vi "Teleop.vi"(10 "Match Info":T1={"Autonomous Elapsed Seconds"=0.0, "TeleOp Elapsed Seconds"=0.0, "Disabled Elapsed Seconds"=0.0, "Visited Autonomous"=FALSE, "Visited TeleOp"=FALSE, "Visited Disabled"=FALSE, "Autonomous Settings"={"Autonomous Style"=enum."Independent", "VI Refnum"=refnum}}, 11 "Call Context":T2) -> ()   [LabVIEW 2015]
doc: "This VI is called for each TeleOp packet received from the DS where the robot is not disabled. It is often used to read from the joysticks and update I/O or to update setpoints for timed control loops. It should complete and return within 20 milliseconds or it may miss DS packets."
uses:
  <vilib>/Rock Robotics/WPI/DriverStation/WPI_DriverStationDerivedRobotMode.ctl
  <vilib>/Rock Robotics/WPI/DriverStation/WPI_DriverStationMatch Info.ctl
  <vilib>/Rock Robotics/WPI/Utilities/WPI_GetSetVariantRefNum.vi
  <vilib>/Rock Robotics/Network Tables/NT Write Boolean Array.vi
  <vilib>/Rock Robotics/Network Tables/NT Write Numeric Array.vi
  <vilib>/Rock Robotics/Network Tables/NT Read Boolean.vi
  <vilib>/Rock Robotics/Network Tables/NT Read Number.vi
  <vilib>/Rock Robotics/Network Tables/NT Write Boolean.vi
  <vilib>/Rock Robotics/Network Tables/NT Write Number.vi
panel:
  out "Low Switch":bool
  out "High Switch":bool
  out "POT Sensor Meter":dbl(knob) scale=78.0..98.0
  out "POT Sensor Value":dbl
  out "Sample Slider 0":dbl(slide) scale=0.0..5.0
  out "Sample Boolean 1":bool
  out "Sample Boolean 0":bool
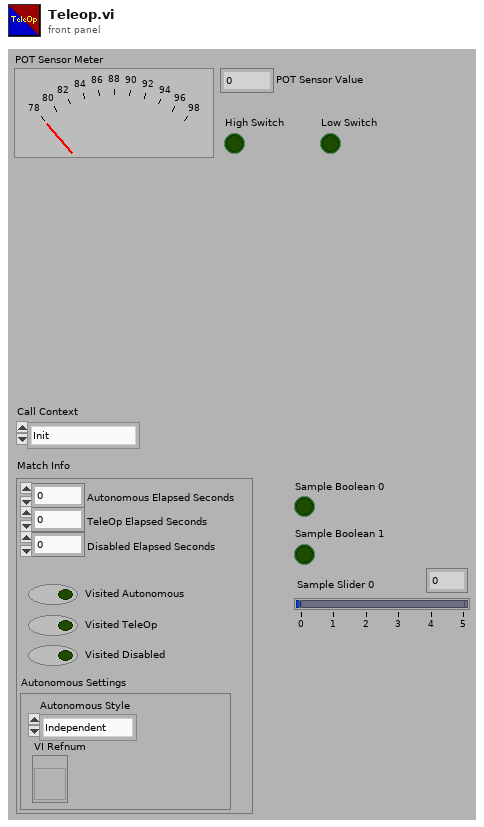
[diagram p1: front panel]
types:
  T1 = typedef "WPI_DriverStationMatch Info.ctl" = cluster{"Autonomous Elapsed Seconds":dbl, "TeleOp Elapsed Seconds":dbl, "Disabled Elapsed Seconds":dbl, "Visited Autonomous":bool, "Visited TeleOp":bool, "Visited Disabled":bool, "Autonomous Settings":cluster{"Autonomous Style":enum16{"Iterative", "Independent"}, "VI Refnum":refnum<vi>}}
  T2 = typedef "WPI_DriverStationDerivedRobotMode.ctl" = enum16{"Init", "Execute", "Stop"}
  T3 = typedef "WPI_JoystickDevRef.ctl" = cluster{"Device":T4}
  T4 = typedef "WPI_JoystickDeviceEnum.ctl" = enum16{"USB 0", "USB 1", "USB 2", "USB 3", "USB 4", "USB 5"}
  T5 = typedef "WPI_SwitchDevRef.ctl" = cluster{"DevStatus":errorcluster, "DIO Channel":T6, "CntIndex":T7, "Normally Closed":bool}
  T6 = typedef "FPGA_DIOChannel.ctl" = enum8{"DIO 0", "DIO 1", "DIO 2", "DIO 3", "DIO 4", "DIO 5", "DIO 6", "DIO 7", "DIO 8", "DIO 9", "DIO MXP 0", "DIO MXP 1", "DIO MXP 2", "DIO MXP 3", "DIO MXP 4", "DIO MXP 5", "DIO MXP 6", "DIO MXP 7", "DIO MXP 8", "DIO MXP 9", "DIO MXP 10", "DIO MXP 11", "DIO MXP 12", "DIO MXP 13", "DIO MXP 14", "DIO MXP 15", "Invalid"}
  T7 = typedef "FPGA_CounterCtrSystemIndex.ctl" = enum8{"Ctr 0", "Ctr 1", "Ctr 2", "Ctr 3", "Ctr 4", "Ctr 5", "Ctr 6", "Ctr 7", "Invalid"}
  T8 = cluster{"Axes[0]":dbl, "Axes[1]":dbl, "Axes[2]":dbl, "Axes[3]":dbl, "Axes[4]":dbl, "Axes[5]":dbl, "Axes[6]":dbl, "Axes[7]":dbl, "Axes[8]":dbl}
  T9 = typedef "WPI_RobotDriveDevRef.ctl" = cluster{"DevStatus":errorcluster, "Motors[]":T10[], "Square Inputs":bool, "Max Output":dbl}
  T10 = typedef "WPI_MotorControlDeviceRef.ctl" = cluster{"DeviceStatus":errorcluster, "Type":T11, "PWM":cluster{"PWM Channel":T12, "DeadBand":T13}, "CAN":cluster{"Device Number":u8, "Control Mode":T14, "Semaphore":T15, "Max Vout":dbl, "TalonSRX Control Mode":T16}, "Invert":bool}
  T11 = typedef "WPI_MotorControlType.ctl" = enum16{"PWM", "CAN", "CANTalonSRX"}
  T12 = typedef "FPGA_DIOPWMChannel.ctl" = enum8{"PWM 0", "PWM 1", "PWM 2", "PWM 3", "PWM 4", "PWM 5", "PWM 6", "PWM 7", "PWM 8", "PWM 9", "PWM MXP 0", "PWM MXP 1", "PWM MXP 2", "PWM MXP 3", "PWM MXP 4", "PWM MXP 5", "PWM MXP 6", "PWM MXP 7", "PWM MXP 8", "PWM MXP 9", "Invalid"}
  T13 = typedef "WPI_PWMDeadband.ctl" = cluster{"Name":string, "maxPositivePwm":i32, "minPositivePwm":i32, "centerPwm":i32, "maxNegativePwm":i32, "minNegativePwm":i32, "angularRange":u16}
  T14 = typedef "WPI_CANJaguar_ControlMode.ctl" = enum8{"Percent VBus", "Current", "Speed", "Position", "Voltage"}
  T15 = typedef "Semaphore RefNum" = refnum<k1>
  T16 = typedef "WPI_CANTalonSRX_APIControlMode.ctl" = enum8{"Percent VBus", "Speed", "Position", "Slave", "Unchanged / Invalid", "Voltage Compensation", "Current", "Motion Profile"}
  T17 = cluster{"Buttons[0]":bool, "Buttons[1]":bool, "Buttons[2]":bool, "Buttons[3]":bool, "Buttons[4]":bool, "Buttons[5]":bool, "Buttons[6]":bool, "Buttons[7]":bool, "Buttons[8]":bool}
  T18 = typedef "WPI_PotentiometerDevRef.ctl" = cluster{"DevStatus":errorcluster, "Analog Channel":T19, "Invert Output":bool}
  T19 = typedef "FPGA_AIChannel.ctl" = enum8{"AI 0", "AI 1", "AI 2", "AI 3", "AI MXP 0", "AI MXP 1", "AI MXP 2", "AI MXP 3", "Invalid"}
  T20 = typedef "WPI_ServoDeviceRef.ctl" = cluster{"DeviceStatus":errorcluster, "PWM Channel":T12, "DeadBand":T13}
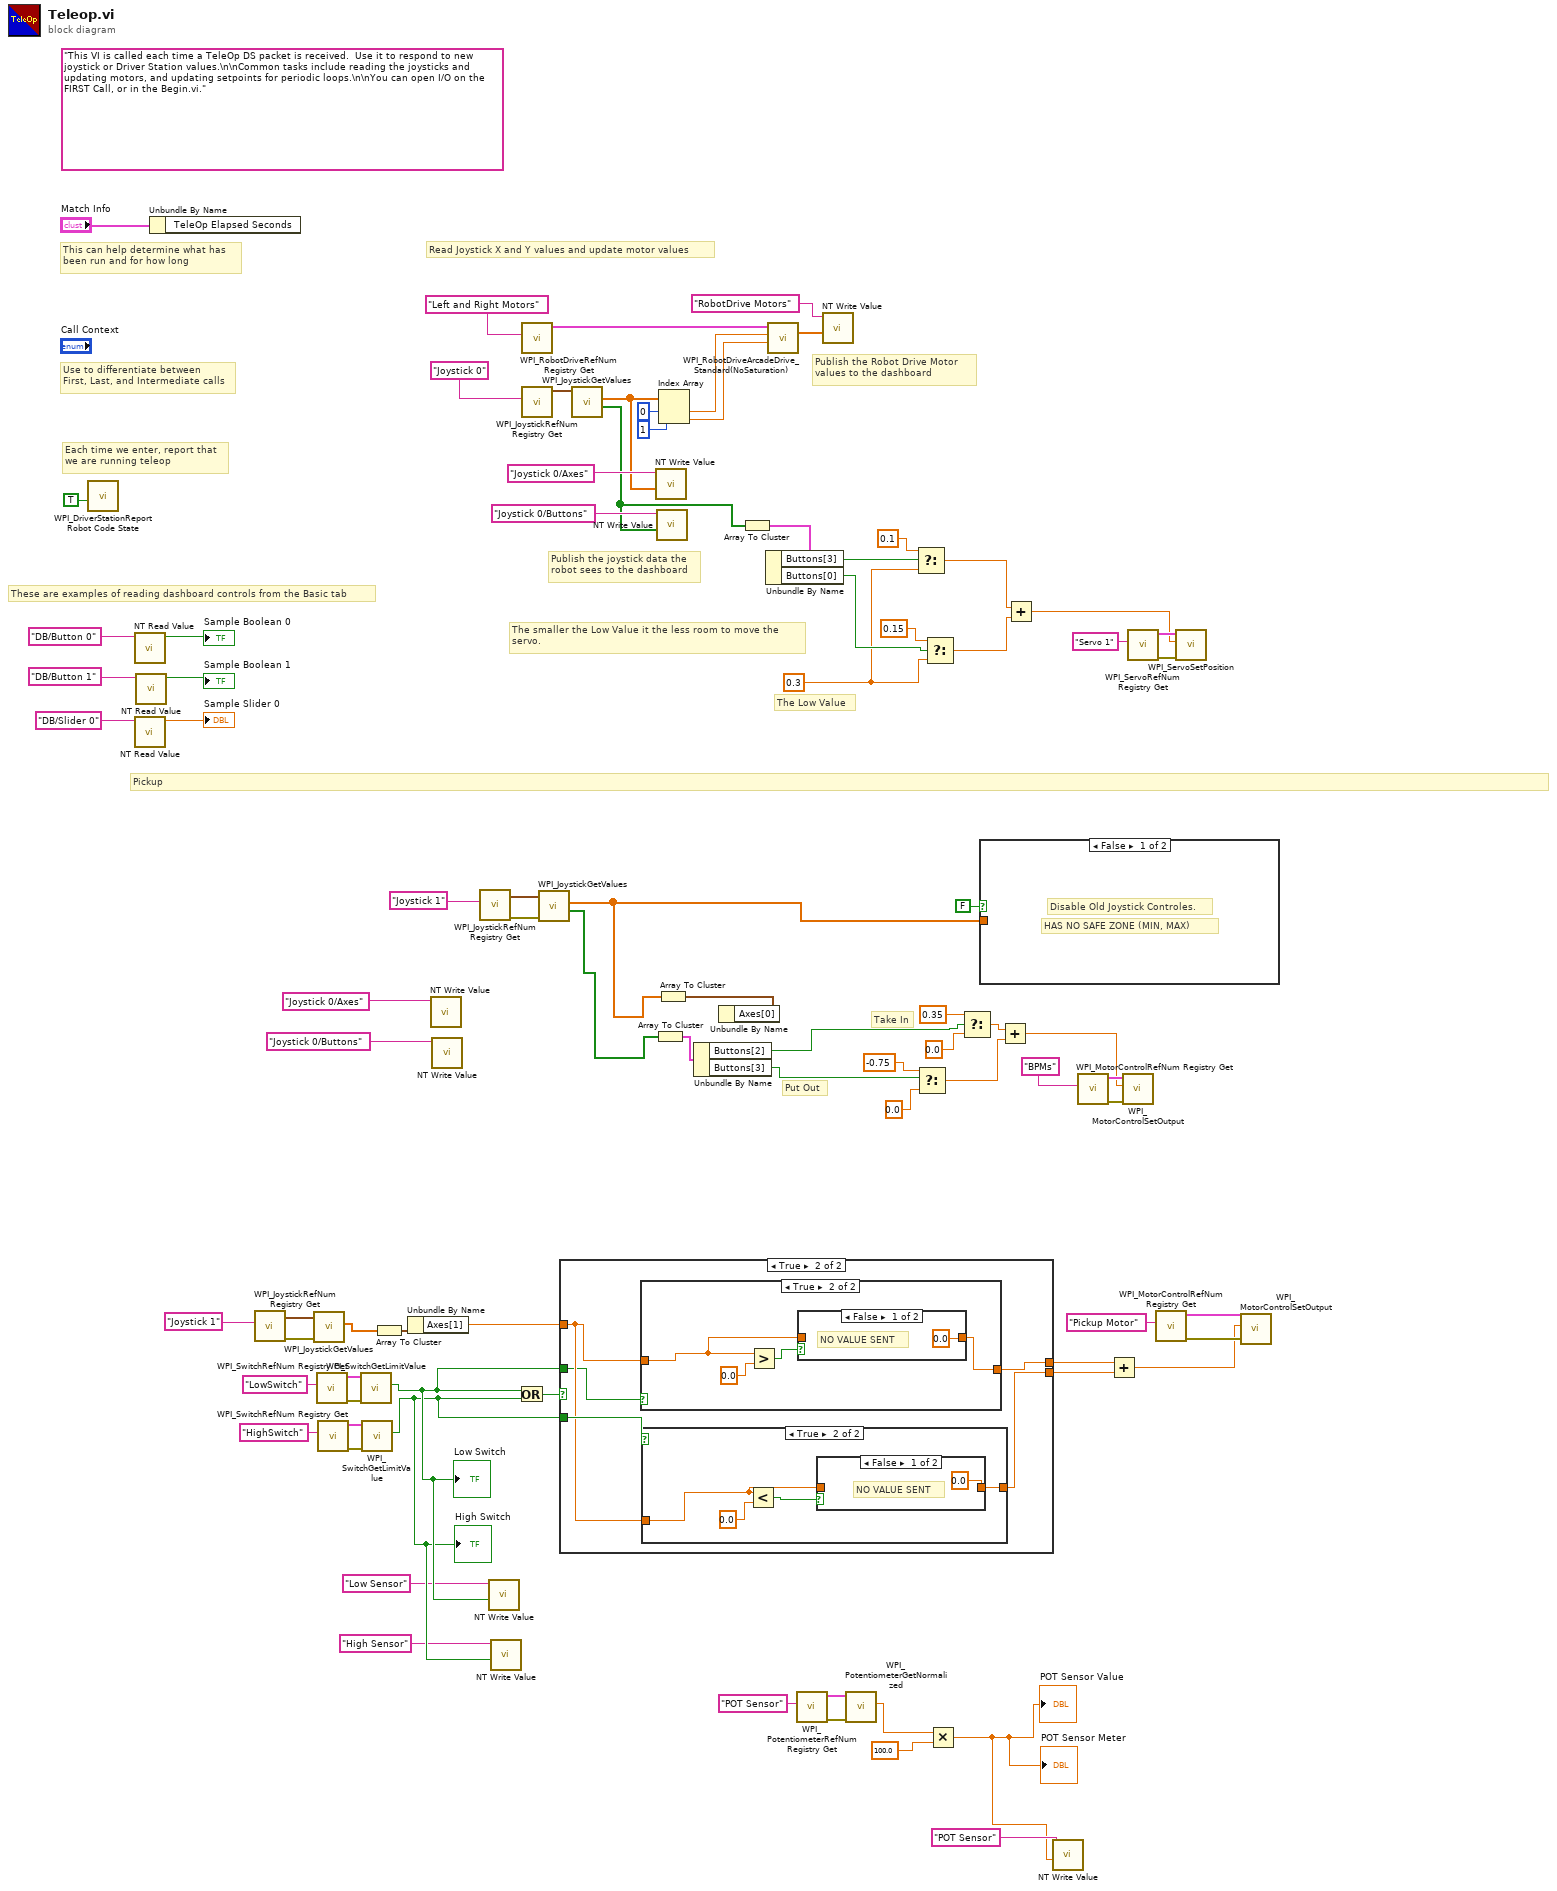
[diagram p0: block diagram]
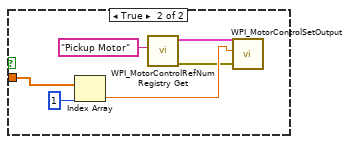
[diagram p2: hidden frame]
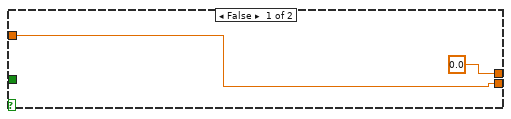
[diagram p3: hidden frame]
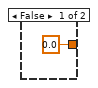
[diagram p4: hidden frame]
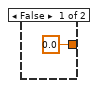
[diagram p6: hidden frame]
diagram:
  w1 = 0.3 ("f")
  (unwired) "This VI is called each time a TeleOp DS packet is received.  Use it to respond to new joystick or Driver Station values.\n\nCommon tasks include reading the joysticks and updating motors, and updating setpoints for periodic loops.\n\nYou can open I/O on the FIRST Call, or in the Begin.vi."
  # "The smaller the Low Value it the less room to move the \nservo."
  # "Put Out"
  # "Take In"
  # "The Low Value"
  # "Pickup"
  # "These are examples of reading dashboard controls from the Basic tab"
  # "Publish the Robot Drive Motor\nvalues to the dashboard"
  # "Publish the joystick data the\nrobot sees to the dashboard"
  # "Each time we enter, report that\nwe are running teleop"
  # "Use to differentiate between\nFirst, Last, and Intermediate calls"
  # "This can help determine what has\nbeen run and for how long"
  # "Read Joystick X and Y values and update motor values"
  n1 = call <vilib>:"WPI_DriverStationReport Robot Code State.vi"("TeleOp"=TRUE ("Autonomous")) -> ()  [unwired: 10 in, 1 out]
  n2 = call-poly <vilib>:"NT Read Value.vi"("Name"="DB/Button 0" ("refnum name")) -> ("Boolean"=→"Sample Boolean 0":bool)  [unwired: 9 in, 1 out]
  n3 = call-poly <vilib>:"NT Read Value.vi"("Name"="DB/Slider 0" ("refnum name")) -> ("Numeric"=→"Sample Slider 0":dbl)  [unwired: 9 in, 1 out]
  n4 = call-poly <vilib>:"NT Read Value.vi"("Name"="DB/Button 1" ("refnum name")) -> ("Boolean"=→"Sample Boolean 1":bool)  [unwired: 9 in, 1 out]
  n5 = Unbundle By Name("Match Info") -> ()  [unwired: 1 out]
  n6 = call <vilib>:"WPI_JoystickRefNum Registry Get.vi"("refnum name"="Joystick 1") -> ("error out"=w27:errorcluster, "JoystickDevRef"=w28:T3)  [unwired: 9 in]
  n7 = call <vilib>:"WPI_JoystickGetValues.vi"("error in (no error)"=w27, "JoystickDevRef"=w28) -> ("Axes"=w26:dbl[])  [unwired: 5 in, 4 out]
  n8 = call <vilib>:"WPI_SwitchRefNum Registry Get.vi"("refnum name"="LowSwitch") -> ("error out"=w34:errorcluster, "SwitchDevRef"=w35:T5)  [unwired: 9 in]
  n9 = call <vilib>:"WPI_SwitchRefNum Registry Get.vi"("refnum name"="HighSwitch") -> ("error out"=w31:errorcluster, "SwitchDevRef"=w32:T5)  [unwired: 9 in]
  n10 = call <vilib>:"WPI_SwitchGetLimitValue.vi"("error in (no error)"=w34, "SwitchDevRef"=w35) -> ("Switch Pressed"=w11:bool)  [unwired: 7 in, 2 out]
  "Low Switch" <- w11
  n11 = call <vilib>:"WPI_SwitchGetLimitValue.vi"("error in (no error)"=w31, "SwitchDevRef"=w32) -> ("Switch Pressed"=w10:bool)  [unwired: 7 in, 2 out]
  "High Switch" <- w10
  n12 = Array To Cluster(array=w26) -> (cluster=w25:T8)
  n13 = Unbundle By Name(w25) -> ("Axes[1]"=w24:dbl)
  n14 = call-poly <vilib>:"NT Write Value.vi"("Name"="Joystick 0/Axes") -> ()  [unwired: 10 in, 1 out]
  n15 = call-poly <vilib>:"NT Write Value.vi"("Name"="Joystick 0/Buttons") -> ()  [unwired: 10 in, 1 out]
  n16 = call <vilib>:"WPI_JoystickRefNum Registry Get.vi"("refnum name"="Joystick 1") -> ("error out"=w63:errorcluster, "JoystickDevRef"=w64:T3)  [unwired: 9 in]
  n17 = call-poly <vilib>:"NT Write Value.vi"("Boolean"=w11, "Name"="Low Sensor") -> ()  [unwired: 9 in, 1 out]
  n18 = call-poly <vilib>:"NT Write Value.vi"("Boolean"=w10, "Name"="High Sensor") -> ()  [unwired: 9 in, 1 out]
  n19 = Or(x=w11, y=w10) -> (x .or. y?=w36:bool)
  n20 = call <vilib>:"WPI_RobotDriveRefNum Registry Get.vi"("refnum name"="Left and Right Motors") -> ("RobotDriveDevRef"=w84:T9)  [unwired: 1 in, 9 out]
  n21 = call <vilib>:"WPI_JoystickRefNum Registry Get.vi"("refnum name"="Joystick 0") -> ("JoystickDevRef"=w81:T3)  [unwired: 1 in, 9 out]
  n22 = call <vilib>:"WPI_JoystickGetValues.vi"("error in (no error)"=w63, "JoystickDevRef"=w64) -> ("Buttons"=w46:bool[], "Axes"=w16:dbl[])  [unwired: 5 in, 3 out]
  n23 = case shown="True" w36 {
    tunnel: w11 -> [_ w91]
    tunnel: w10 -> [_ w93]
    tunnel: w24 -> [w87 w92]
    tunnel: [0.0 ("Axes[1]") w90] -> w19
    tunnel: [w87 w89] -> w18
    frame False {
    }
    frame True {
      n24 = case shown="True" w91 {
        tunnel: w92 -> [_ w103]
        tunnel: [0.0 ("Axes[1]") w102] -> w90
        frame False {
        }
        frame True {
          n25 = Greater?(x=w103, y=0.0) -> (0:w104:bool)
          n26 = case shown="False" w104 {
            tunnel: [0.0 ("Axes[1]") w107] -> w102
            tunnel: w103 -> [_ w107]
            frame False {
              # "NO VALUE SENT"
            }
            frame True {
            }
          }
        }
      }
      n27 = case shown="True" w93 {
        tunnel: w92 -> [_ w95]
        tunnel: [0.0 ("Axes[1]") w96] -> w89
        frame False {
        }
        frame True {
          n28 = Less?(x=w95, y=0.0) -> (x < y?=w97:bool)
          n29 = case shown="False" w97 {
            tunnel: [0.0 ("Axes[1]") w100] -> w96
            tunnel: w95 -> [_ w100]
            frame False {
              # "NO VALUE SENT"
            }
            frame True {
            }
          }
        }
      }
    }
  }
  n30 = call <vilib>:"WPI_JoystickGetValues.vi"("JoystickDevRef"=w81) -> ("Buttons"=w41:bool[], "Axes"=w76:dbl[])  [unwired: 6 in, 3 out]
  n31 = Array To Cluster(array=w46) -> (cluster=w44:T17)
  n32 = call-poly <vilib>:"NT Write Value.vi"("Numeric Array"=w76, "Name"="Joystick 0/Axes") -> ()  [unwired: 9 in, 1 out]
  n33 = call-poly <vilib>:"NT Write Value.vi"("Boolean Array"=w41, "Name"="Joystick 0/Buttons") -> ()  [unwired: 9 in, 1 out]
  n34 = Array To Cluster(array=w16) -> (cluster=w45:T8)
  n35 = Index Array(array=w76, index #1=0 ("index"), index #2=1 ("index")) -> (element #1=w83:dbl, element #2=w79:dbl)
  n36 = Unbundle By Name(w44) -> ("Buttons[2]"=w43:bool, "Buttons[3]"=w42:bool)
  n37 = Unbundle By Name(w45) -> ()  [unwired: 1 out]
  n38 = Array To Cluster(array=w41) -> (cluster=w40:T17)
  n39 = Unbundle By Name(w40) -> ("Buttons[3]"=w39:bool, "Buttons[0]"=w37:bool)
  n40 = call <vilib>:"WPI_RobotDriveArcadeDrive_Standard(NoSaturation).vi"("Y axis value"=w79, "X axis value"=w83, "RobotDriveDevRef"=w84) -> ("Motor Values"=w69:dbl[])  [unwired: 1 in, 7 out]
  n41 = call <vilib>:"WPI_PotentiometerRefNum Registry Get.vi"("refnum name"="POT Sensor") -> ("error out"=w15:errorcluster, "PotDevRef"=w14:T18)  [unwired: 9 in]
  n42 = call-poly <vilib>:"NT Write Value.vi"("Numeric Array"=w69, "Name"="RobotDrive Motors") -> ()  [unwired: 9 in, 1 out]
  n43 = call <vilib>:"WPI_PotentiometerGetNormalized.vi"("error in"=w15, "PotDevRef"=w14) -> ("Normalized Value"=w7:dbl)  [unwired: 7 in, 2 out]
  n44 = Select(t=0.1, s=w39, f=w1) -> (s? t:f=w4:dbl)
  n45 = Select(t=-0.75, s=w42, f=0.0) -> (s? t:f=w54:dbl)
  n46 = Select(t=0.15, s=w37, f=w1) -> (s? t:f=w3:dbl)
  n47 = Multiply(x=w7, y=100.0) -> (x*y=w5:dbl)
  "POT Sensor Value" <- w5
  "POT Sensor Meter" <- w5
  n48 = Select(t=0.35, s=w43, f=0.0) -> (s? t:f=w55:dbl)
  n49 = case shown="False" FALSE {
    tunnel: w16 -> [_ w108]
    frame False {
      # "HAS NO SAFE ZONE (MIN, MAX)"
      # "Disable Old Joystick Controles."
    }
    frame True {
      n50 = Index Array(array=w108, index=1) -> (element=w112:dbl)
      n51 = call <vilib>:"WPI_MotorControlRefNum Registry Get.vi"("refnum name"="Pickup Motor") -> ("error out"=w109:errorcluster, "MotorControlDevRef"=w110:T10)  [unwired: 9 in]
      n52 = call <vilib>:"WPI_MotorControlSetOutput.vi"("error in (no error)"=w109, "Output"=w112, "MotorControlDevRef"=w110) -> ()  [unwired: 6 in, 3 out]
    }
  }
  n53 = Add(x=w55, y=w54) -> (x+y=w53:dbl)
  n54 = Add(x=w4, y=w3) -> (x+y=w2:dbl)
  n55 = call-poly <vilib>:"NT Write Value.vi"("Numeric"=w5, "Name"="POT Sensor") -> ()  [unwired: 9 in, 1 out]
  n56 = call <vilib>:"WPI_MotorControlRefNum Registry Get.vi"("refnum name"="BPMs") -> ("error out"=w61:errorcluster, "MotorControlDevRef"=w62:T10)  [unwired: 9 in]
  n57 = Add(x=w19, y=w18) -> (x+y=w20:dbl)
  n58 = call <vilib>:"WPI_MotorControlSetOutput.vi"("error in (no error)"=w61, "Output"=w53, "MotorControlDevRef"=w62) -> ()  [unwired: 6 in, 3 out]
  n59 = call <vilib>:"WPI_ServoRefNum Registry Get.vi"("refnum name"="Servo 1") -> ("error out"=w51:errorcluster, "ServoDeviceRef"=w50:T20)  [unwired: 9 in]
  n60 = call <vilib>:"WPI_MotorControlRefNum Registry Get.vi"("refnum name"="Pickup Motor") -> ("error out"=w23:errorcluster, "MotorControlDevRef"=w22:T10)  [unwired: 9 in]
  n61 = call <vilib>:"WPI_ServoSetPosition.vi"("error in (no error)"=w51, "Position"=w2, "ServoDeviceRef"=w50) -> ()  [unwired: 7 in, 2 out]
  n62 = call <vilib>:"WPI_MotorControlSetOutput.vi"("error in (no error)"=w23, "Output"=w20, "MotorControlDevRef"=w22) -> ()  [unwired: 6 in, 3 out]
